vi "Init.vi"(8 "error in (no error)":errorcluster, 11 "Index":i32) -> (0 "error out":errorcluster, 3 "Device out":refnum<class "Device.lvclass">)   [LabVIEW 2020, in "RTL-SDR.lvlib" / "Device.lvclass"]
uses:
  Device.lvclass
  Device.lvclass/Device.ctl
  lib/librtlsdr.dll
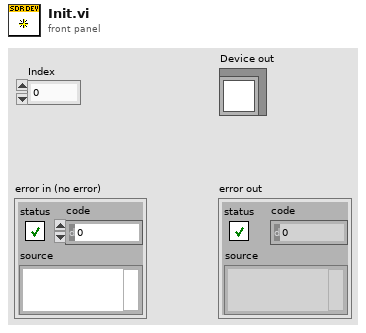
[diagram p1: front panel]
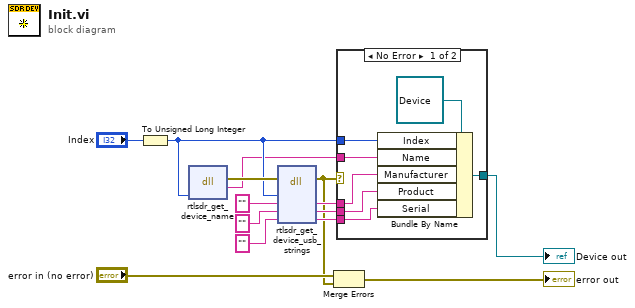
[diagram p0: block diagram]
diagram:
  n1 = To Unsigned Long Integer(number="Index") -> (unsigned 32bit integer=w7:u32)
  n2 = dll-call lib="C:/dev/IlluminatedG/rtl-sdr/lib/librtlsdr.dll" fn="rtlsdr_get_device_name"("index"=w7) -> (error out=w12:errorcluster, "return type"=w6:string)  [unwired: 4 in, 1 out]
  n3 = dll-call lib="C:/dev/IlluminatedG/rtl-sdr/lib/librtlsdr.dll" fn="rtlsdr_get_device_usb_strings"(error in=w12, "index"=w7, "manufact"="", "product"="" ("manufact"), "serial"="" ("manufact")) -> (error out=w1:errorcluster, "manufact"=w5:string, "product"=w4:string, "serial"=w3:string)  [unwired: 4 in, 1 out]
  n4 = Merge Errors("error in (no error)", w1) -> (→"error out":errorcluster)
  n5 = case shown="No Error" w1 {
    tunnel: [w20 _] -> w8
    tunnel: w7 -> [w19 _]
    tunnel: w6 -> [w18 _]
    tunnel: w5 -> [w17 _]
    tunnel: w4 -> [w16 _]
    tunnel: w3 -> [w15 _]
    frame No Error {
      n6 = Bundle By Name(cluster=refnum<class "Device.lvclass"> refnum ("Device in"), "Index"=w19, "Name"=w18, "Manufacturer"=w17, "Product"=w16, "Serial"=w15) -> (w20:refnum<class "Device.lvclass">)
    }
    frame Error {
    }
  }
  "Device out" <- w8
